vi "SV TDMS Read Even-Angle Signal (N Ch).vi"(0 "tdms file":refnum<k34>, 5 "group name in":string="Even-Angle_Signal", 7 "channel names in":string[](array[string]), 11 "error in":errorcluster) -> (4 "tdms file out":refnum<k34>, 6 "group name out":string, 8 "channel names out":string[](array[string]), 10 "even-angle signals":cluster{"r0":dbl, "dr":dbl, "Y":dbl[]}[](array[cluster]) {"r0" format="%.2p"; "dr" format="%.2p"; "Y" format="%.2f"}, 12 "even-angle position info":T1, 13 "even-angle channel info":T2[](array[typedef]) {"channel info"."pregain" format="%.2f"; "channel info"."weighting filter" items=["Linear", "A-weighting", "B-weighting", "C-weighting", "ITU-R 468-4", "Dolby", "CCITT", "C-message", "Wb", "Wc", "Wd", "We", "Wf", "Wh", "Wj", "Wk", "Wm", "AES17 20 kHz lowpass", "AES17 40 kHz lowpass", "AES17 20 kHz highpass", "AES17 40 kHz highpass"]; "channel info"."dB reference" format="%^.1e"; "channel info"."engineering units" items=["custom..."=0, "V"=1, "A"=21, "C"=30, "pC"=31, "s"=32, "-"=29, "Pa"=2, "N"=20, "g"=3, "m/s^2"=4, "m/s"=5, "m"=6, "mm/s"=12, "mm"=13, "micron/s"=14, "micron"=15, "in/s^2"=7, "in/s"=8, "in"=9, "mil/s"=10, "mil"=11, "rad/s^2"=16, "rad/s"=17, "rad"=18, "deg/s^2"=26, "deg/s"=27, "deg"=28, "RPM"=22, "cycle/s^2"=23, "Hz"=24, "cycle"=25, "strain"=19]; "channel info"."sensor sensitivity" format="%#_5f"}, 15 "error out":errorcluster)   [LabVIEW 2017]
doc: "Reads the specified .tdms file and returns data in a format specific to the polymorphic instance selected."
uses:
  <vilib>/addons/_NISVFA/_Shared subVIs/Controls/svc_Resampled Channel Info.ctl
  <vilib>/addons/_NISVFA/_Shared subVIs/Controls/svc_Channel Info.ctl
  <vilib>/addons/_NISVFA/_Shared subVIs/Controls/svc_Engineering Units Text Ring.ctl
  <vilib>/addons/_NISVFA/_Shared subVIs/Controls/svc_Weighting Filter Text Ring.ctl
  <vilib>/addons/_NISVFA/_Shared subVIs/Controls/svc_Position Info.ctl
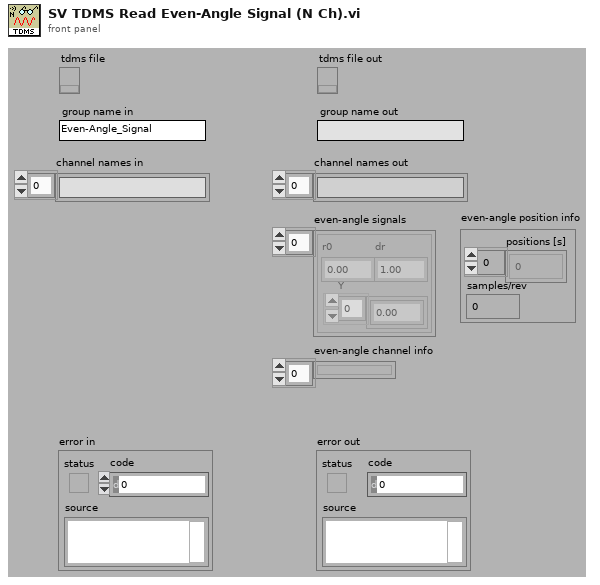
[diagram p1: front panel]
types:
  T1 = typedef "svc_Position Info.ctl" = cluster{"positions [s]":dbl[], "samples/rev":dbl}
  T2 = typedef "svc_Resampled Channel Info.ctl" = cluster{"channel name":string, "description":string, " channel info":T3}
  T3 = typedef "svc_Channel Info.ctl" = cluster{"sensor sensitivity":dbl, "engineering units":T4, "dB reference":dbl, "custom label":string, "weighting filter":T5, "pregain":dbl}
  T4 = typedef "svc_Engineering Units Text Ring.ctl" = u16
  T5 = typedef "svc_Weighting Filter Text Ring.ctl" = u16
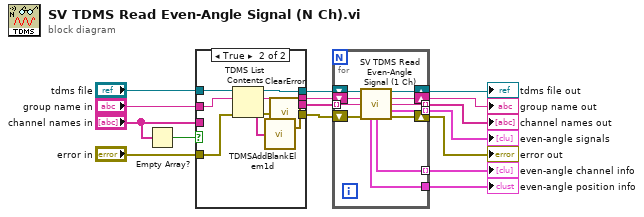
[diagram p0: block diagram]
diagram:
  n1 = Empty Array?(array="channel names in") -> (empty?=w15:bool)
  n2 = case shown="True" w15 {
    tunnel: "tdms file" -> [w20 w29]
    tunnel: [w20 w28] -> w13
    tunnel: "group name in" -> [w19 w27]
    tunnel: [w19 w26] -> w11
    tunnel: [w18 w25] -> w10
    tunnel: "channel names in" -> [w18 _]
    tunnel: [w17 w24] -> w6
    tunnel: "error in" -> [w17 w23]
    frame False {
    }
    frame True {
      n3 = TDMS List Contents(4:w23, 6:w27, 7:w29) -> (0:w21:errorcluster, 1:w22:string[], 2:w26:string, 3:w28:refnum<k34>)
      n4 = call <vilib>:"TDMSAddBlankElem1d.vi"("input string array"=w22) -> ("output string array with blank element at the beginning"=w25:string[])
      n5 = call <vilib>:"ClearError.vi"("error in (no error)"=w21) -> ("error out"=w24:errorcluster)
    }
  }
  n6 = for {
    tunnel: w10 -> [w37] mode=indexing
    shift-right: [w40] -> w16
    shift-left: w13 -> [w39]
    shift-right: [w36] -> w8
    shift-left: w11 -> [w38]
    tunnel: [w35] -> w7 mode=indexing
    shift-right: [w33] -> w4
    shift-left: w6 -> [w34]
    tunnel: [w32] -> w3 mode=indexing
    tunnel: [w31] -> w2 mode=indexing
    tunnel: [w30] -> w1
    n7 = call <vilib>:"SV TDMS Read Even-Angle Signal (1 Ch).vi"("tdms file"=w39, "group name in"=w38, "channel name in"=w37, "error in"=w34) -> ("tdms file out"=w40:refnum<k34>, "group name out"=w36:string, "channel name out"=w35:string, "even-angle signal"=w32:cluster{"r0":dbl, "dr":dbl, "Y":dbl[]}, "even-angle position info"=w30:T1, "even-angle channel info"=w31:T2, "error out"=w33:errorcluster)  [unwired: 5 in]
  }
  "even-angle channel info" <- w2
  "error out" <- w4
  "tdms file out" <- w16
  "even-angle signals" <- w3
  "group name out" <- w8
  "channel names out" <- w7
  "even-angle position info" <- w1
